vi "QueryBCMOut.vi"(8 "error in (no error)":errorcluster, 11 "COM Port":refnum<visa-resource-name>="COM3") -> (0 "error out":errorcluster, 2 "BCMOut":i32, 3 "COM Port Out":refnum<visa-resource-name>="COM3")   [LabVIEW 2020]
panel:
  in  "Ucal":dbl
  in  "Qcal":dbl
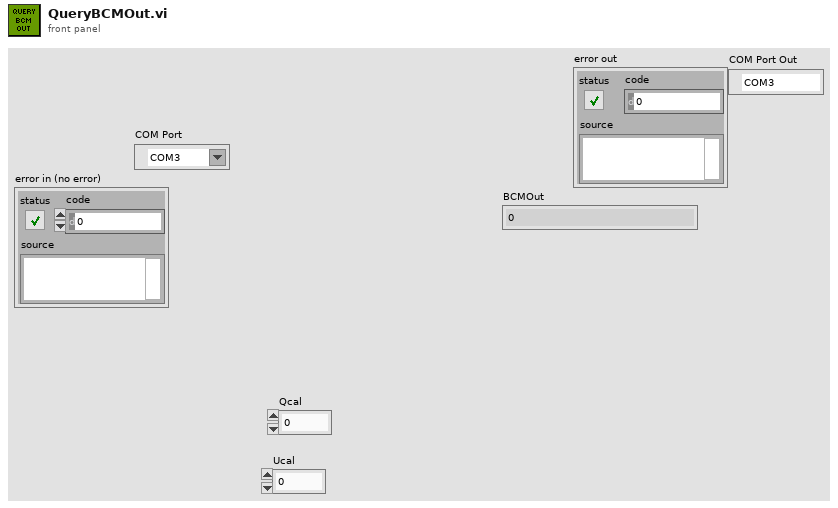
[diagram p1: front panel]
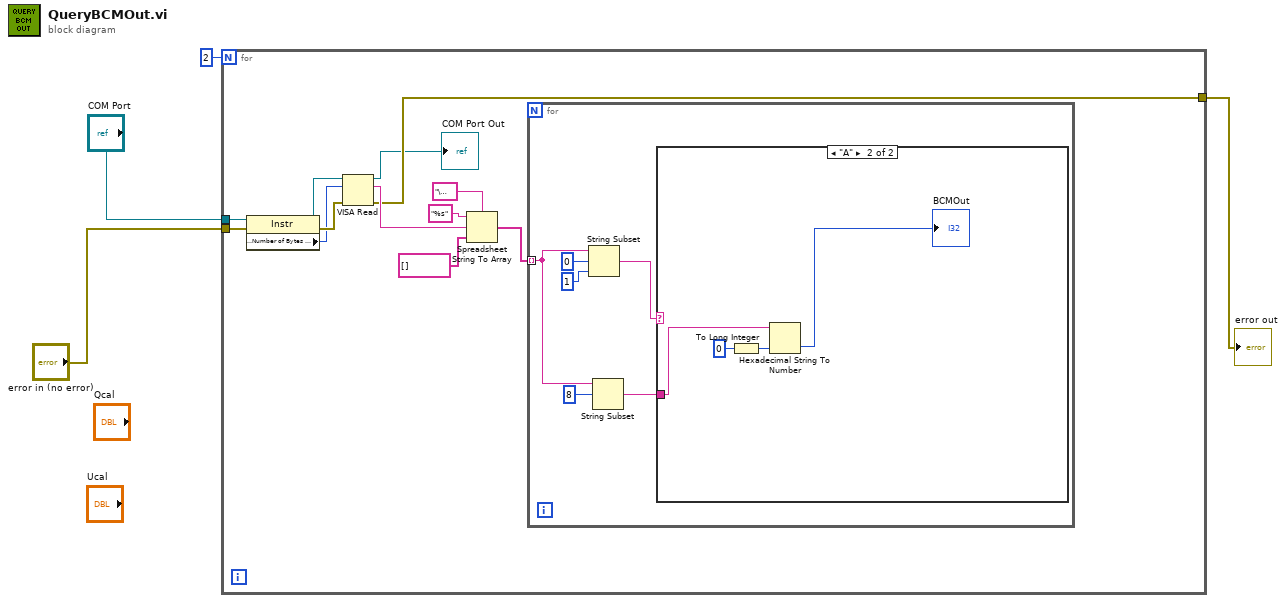
[diagram p0: block diagram]
diagram:
  n1 = for {
    N: 2 -> [_]
    tunnel: "COM Port" -> [w16]
    tunnel: "error in (no error)" -> [w15]
    tunnel: [w6] -> w1
    n2 = property class="Instr"(reference=w16, error in=w15) -> (reference out=w10:refnum<visa-resource-name>, error out=w9:errorcluster, "Serial Settings:Number of Bytes at Serial Port"=w8:u32)
    n3 = VISA Read(VISA resource name=w10, byte count=w8, error in (no error)=w9) -> (VISA resource name out=→"COM Port Out":refnum<visa-resource-name>, read buffer=w13:string, error out=w6:errorcluster)  [unwired: 1 out]
    n4 = Spreadsheet String To Array(delimiter (Tab)="\u0000", format string="%s", spreadsheet string=w13, array type (2D Dbl)=string[] []) -> (array=w7:string[])
    n5 = for {
      tunnel: w7 -> [w19] mode=indexing
      n6 = String Subset(string=w19, offset (0)=0 ("index"), length (rest)=1 ("length")) -> (substring=w18:string)
      n7 = String Subset(string=w19, offset (0)=8 ("index")) -> (substring=w17:string)  [unwired: 1 in]
      n8 = case shown="\"A\"" w18 {
        tunnel: w17 -> [_ w24]
        frame "False", Default {
        }
        frame "A" {
          n9 = To Long Integer(number=0 ("default (0 U32)")) -> (32bit integer=w26:i32)
          n10 = Hexadecimal String To Number(string=w24, default (0uL)=w26) -> (number=→"BCMOut":i32)  [unwired: 1 in, 1 out]
        }
      }
    }
  }
  "error out" <- w1
